vi "DP Waveform Averager PXI.vi"(0 "DataAcq":T3, 1 "DP Freqs":T2, 7 "iLevel":i32, 11 "error in":errorcluster, 12 "Abort":refnum<vi>, 13 "Reject Ref":T1) -> (4 "Error?":bool, 6 "Ave Wave":dbl[](graph), 8 "Averaged Spectrum (Vrms)":dbl[](array[numeric]), 10 "Phase spectrum":dbl[](array[numeric]), 14 "waveform cluster":cluster{i32, "dx":dbl, "Array":dbl[]}, 15 "error out":errorcluster)   [LabVIEW 2020]
uses:
  afcfbcde-8fef-4170-88b9-8379dbc42e1a.vi
  Typedefs/DP-Runtime State.ctl
  Typedefs/DP-Freqs.ctl
  Typedefs/DP-Rejection Settings.ctl
  Typedefs/DP-Rejection Settings Refnum.ctl
panel:
  out "# Spectra":i32
  out "# Waves":i32
  out "Spectrum":cluster{dbl, "dx":dbl, "Y":dbl[]}(graph)
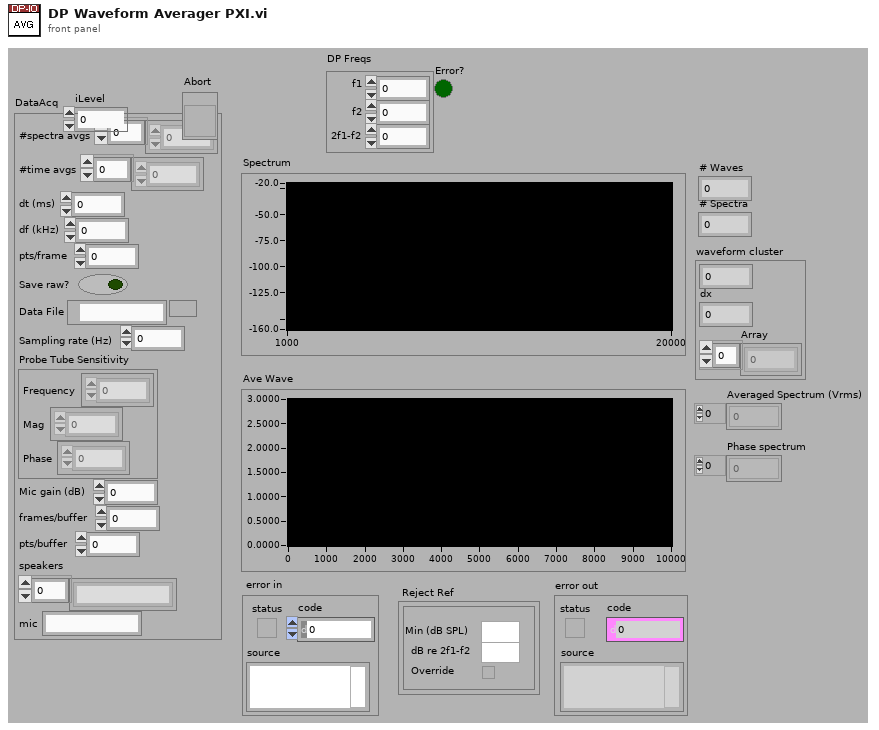
[diagram p1: front panel]
types:
  T1 = typedef "DP-Rejection Settings Refnum.ctl" = refnum<vi>
  T2 = typedef "DP-Freqs.ctl" = cluster{"f1":dbl, "f2":dbl, "2f1-f2":dbl}
  T3 = typedef "DP-Runtime State.ctl" = cluster{"#spectra avgs":i32[], "#time avgs":i32[], "dt (ms)":dbl, "df (kHz)":dbl, "pts/frame":i32, "Save raw?":bool, "Data File":path, "Sampling rate (Hz)":dbl, "Probe Tube Sensitivity":cluster{"Frequency":dbl[], "Mag":dbl[], "Phase":dbl[]}, "Mic gain (dB)":dbl, "frames/buffer":i32, "pts/buffer":i32, "speakers":string[], "mic":string}
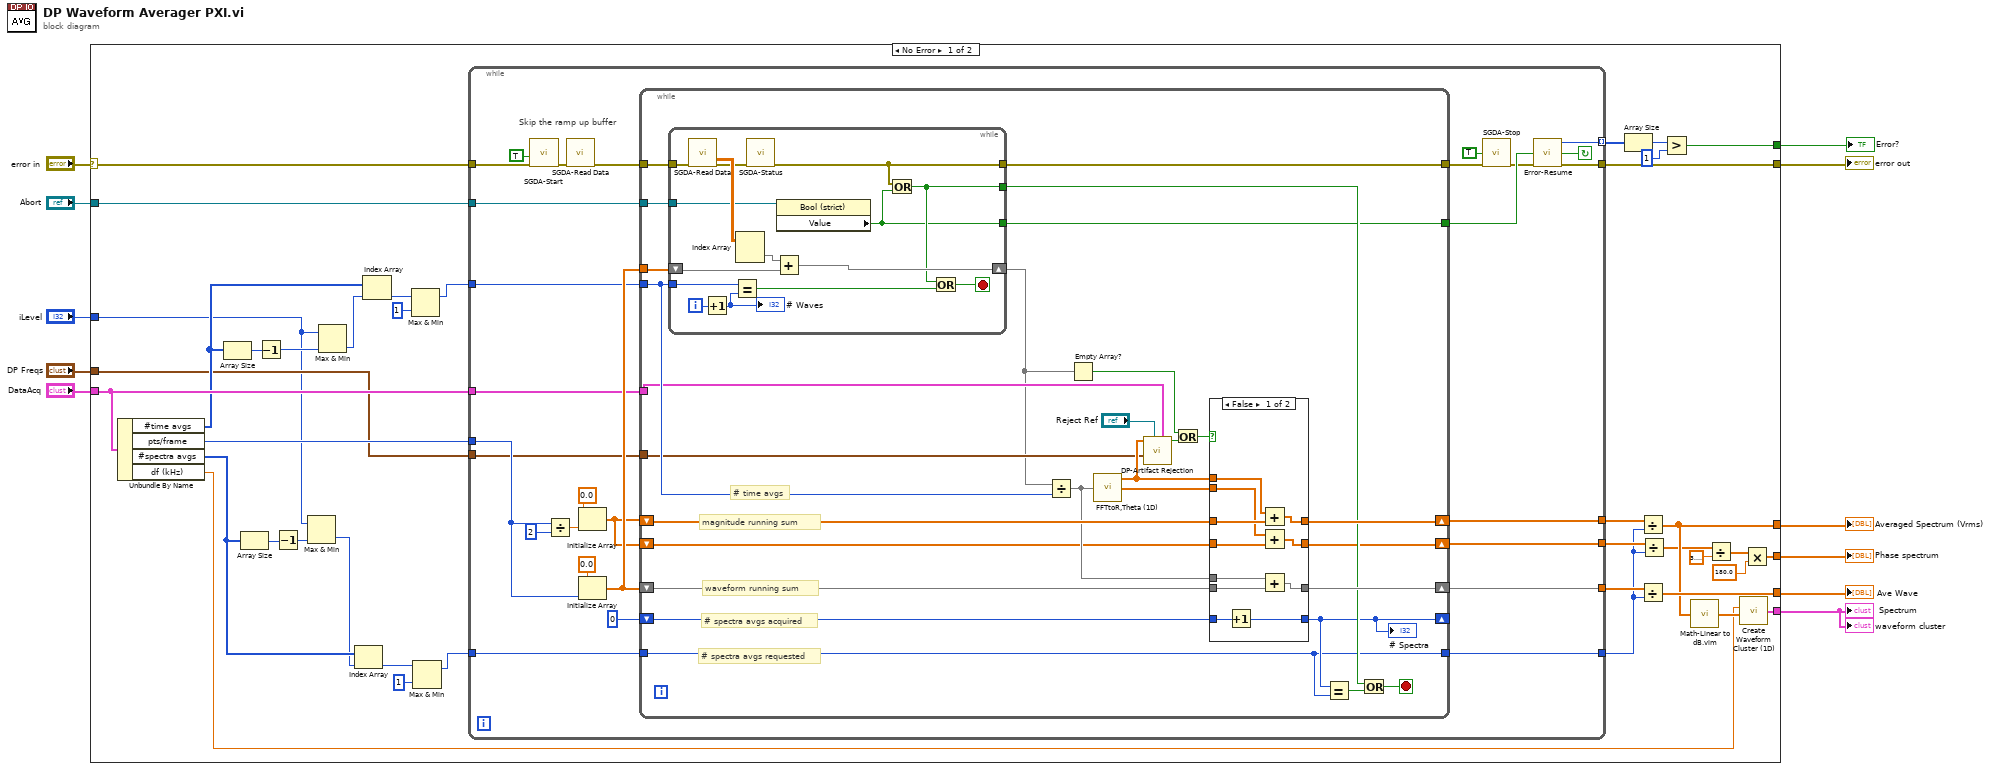
[diagram p0: block diagram]
diagram:
  n1 = case shown="No Error" "error in" {
    selector: "error in" -> [w28 w137]
    tunnel: [w48 _] -> w11
    tunnel: [w47 _] -> w10
    tunnel: [w43 _] -> w9
    tunnel: "Abort" -> [w42 _]
    tunnel: [w37 _] -> w7
    tunnel: "DataAcq" -> [w34 _]
    tunnel: [w33 w137] -> w5
    tunnel: [w29 _] -> w4
    tunnel: "iLevel" -> [w19 _]
    tunnel: "DP Freqs" -> [w21 _]
    frame No Error {
      n2 = Unbundle By Name(w34) -> ("#time avgs"=w27:i32[], "pts/frame"=w45:i32, "#spectra avgs"=w20:i32[], "df (kHz)"=w44:dbl)
      n3 = Array Size(array=w27) -> (size(s)=w26:i32)
      n4 = Array Size(array=w20) -> (size(s)=w23:i32)
      n5 = Decrement(x=w26) -> (x-1=w25:i32)
      n6 = Decrement(x=w23) -> (x-1=w22:i32)
      n7 = Max & Min(x=w19, y=w22) -> (min(x,y)=w18:i32)  [unwired: 1 out]
      n8 = Max & Min(x=w19, y=w25) -> (min(x,y)=w24:i32)  [unwired: 1 out]
      n9 = Index Array(array=w20, index=w18) -> (element=w13:i32)
      n10 = Index Array(array=w27, index=w24) -> (element=w17:i32)
      n11 = Max & Min(x=w17, y=1) -> (max(x,y)=w16:i32)  [unwired: 1 out]
      n12 = Max & Min(x=w13, y=1) -> (max(x,y)=w12:i32)  [unwired: 1 out]
      n13 = while {
        tunnel: [w78] -> w50
        tunnel: [w76] -> w49
        tunnel: [w56] -> w33
        tunnel: w16 -> [w70]
        tunnel: w45 -> [w69]
        tunnel: w42 -> [w68]
        tunnel: w28 -> [w67]
        tunnel: [w62] -> w41
        tunnel: w12 -> [w60]
        tunnel: [w59] -> w35
        tunnel: w21 -> [w58]
        tunnel: w34 -> [w57]
        tunnel: [w53] -> w32 mode=indexing
        stop <- w55 continue-if-true
        # "Skip the ramp up buffer"
        n14 = call "SGDA-Start.vi"("error in (no error)"=w67, "wait for DAQ? (F)"=TRUE) -> ("error out"=w65:errorcluster)  [unwired: 5 in]
        n15 = Divide(x=w69, y=2) -> (x/y=w71:dbl)
        n16 = call "SGDA-Read Data.vi"("error in (no error)"=w65) -> ("error out"=w66:errorcluster)  [unwired: 13 in, 1 out]
        n17 = Initialize Array(0.0, w71) -> (w63:dbl[])
        n18 = Initialize Array(0.0, w69) -> (w74:dbl[])
        n19 = while {
          tunnel: w70 -> [w100]
          shift-right: [w105] -> w78
          shift-left: w63 -> [w106]
          shift-right: [w103] -> w76
          shift-left: w74 -> [w104]
          tunnel: w74 -> [w101]
          tunnel: w66 -> [w102]
          tunnel: [w82] -> w75
          tunnel: w68 -> [w95]
          shift-right: [w94] -> w62
          shift-left: w63 -> [w92]
          shift-right: [w88] -> _
          shift-left: 0 -> [w89]
          tunnel: w60 -> [w87]
          tunnel: [w87] -> w59
          tunnel: w58 -> [w86]
          tunnel: w57 -> [w84]
          tunnel: [w83] -> w54
          stop <- w97 stop-if-true
          # "# spectra avgs acquired"
          # "# spectra avgs requested"
          # "# time avgs"
          # "waveform running sum"
          # "magnitude running sum"
          n20 = while {
            shift-right: [w133] -> w80
            shift-left: w101 -> [w134]
            tunnel: w100 -> [w132]
            tunnel: [w126] -> w98
            tunnel: w102 -> [w135]
            tunnel: [w122] -> w82
            tunnel: w95 -> [w125]
            tunnel: [w124] -> w83
            i -> [w131]
            stop <- w128 stop-if-true
            n21 = call "SGDA-Read Data.vi"("error in (no error)"=w135) -> ("AI Waveforms"=w136:dbl[][], "error out"=w123:errorcluster)  [unwired: 13 in]
            n22 = Increment(x=w131) -> (x+1=w130:i32)
            "# Waves" <- w130
            n23 = Equal?(x=w132, y=w130) -> (x = y?=w127:bool)
            n24 = Index Array(array=w136) -> (element=w129:dbl[])  [unwired: 2 in]
            n25 = call "SGDA-Status.vi"("error in (no error)"=w123) -> ("error out"=w122:errorcluster)  [unwired: 14 in]
            n26 = Add(x=w129, y=w134) -> (x+y=w133:dbl[])
            n27 = property class="Bool (strict)"(reference=w125) -> ("Value"=w124:bool)  [unwired: 1 in, 2 out]
            n28 = Or(x=w122, y=w124) -> (x .or. y?=w126:bool)
            n29 = Or(x=w126, y=w127) -> (x .or. y?=w128:bool)
          }
          n30 = Divide(x=w80, y=w100) -> (x/y=w99:dbl[])
          n31 = Empty Array?(array=w80) -> (empty?=w79:bool)
          n32 = call "FFTtoR,Theta (1D).VI"("X"=w99) -> ("+Freq. Mag of FFT"=w91:dbl[], "+Freq Theta of FFT"=w93:dbl[])  [unwired: 1 in]
          n33 = call "DP-Artifact Rejection.vi"("DataAcq"=w84, "Reject Ref"="Reject Ref", "DP Freqs"=w86, "Magnitude (Vrms)"=w91) -> ("Reject?"=w90:bool)  [unwired: 7 in]
          n34 = Or(x=w79, y=w90) -> (x .or. y?=w81:bool)
          n35 = case shown="False" w81 {
            tunnel: w106 -> [w117 w121]
            tunnel: [w116 w121] -> w105
            tunnel: w104 -> [w115 w119]
            tunnel: [w114 w119] -> w103
            tunnel: w99 -> [w113 _]
            tunnel: [w112 w120] -> w94
            tunnel: w93 -> [w111 _]
            tunnel: w92 -> [w110 w120]
            tunnel: w91 -> [w109 _]
            tunnel: w89 -> [w108 w118]
            tunnel: [w107 w118] -> w88
            frame False {
              n36 = Increment(x=w108) -> (x+1=w107:i32)
              n37 = Add(x=w109, y=w117) -> (x+y=w116:dbl[])
              n38 = Add(x=w111, y=w110) -> (x+y=w112:dbl[])
              n39 = Add(x=w113, y=w115) -> (x+y=w114:dbl[])
            }
            frame True {
            }
          }
          "# Spectra" <- w88
          n40 = Equal?(x=w88, y=w87) -> (x = y?=w96:bool)
          n41 = Or(x=w98, y=w96) -> (x .or. y?=w97:bool)
        }
        n42 = call "SGDA-Stop.vi"("Clear ActiveX (F)"=TRUE, "error in (no error)"=w75) -> ("error out"=w52:errorcluster)  [unwired: 13 in]
        n43 = call "Error-Resume.vi"("Abort"=w54, "error in (no error)"=w52) -> ("code"=w53:i32, "Resume?"=w55:bool, "error out"=w56:errorcluster)  [unwired: 11 in]
      }
      n44 = Array Size(array=w32) -> (size(s)=w31:i32)
      n45 = Divide(x=w50, y=w35) -> (x/y=w47:dbl[])
      n46 = Divide(x=w49, y=w35) -> (x/y=w48:dbl[])
      n47 = Divide(x=w41, y=w35) -> (x/y=w40:dbl[])
      n48 = Greater?(x=w31, y=1) -> (0:w29:bool)
      n49 = call "Math-Linear to dB.vim"("linear"=w47) -> ("dB"=w46:dbl[])
      n50 = Divide(x=w40, y=3.141592653589793) -> (x/y=w39:dbl[])
      n51 = call "Create Waveform Cluster (1D).vi"("dx"=w44, "Y"=w46) -> ("waveform cluster"=w43:cluster{dbl, "dx":dbl, "Y":dbl[]})  [unwired: 3 in]
      n52 = Multiply(x=w39, y=180.0) -> (x*y=w37:dbl[])
    }
    frame Error {
    }
  }
  "Spectrum" <- w9
  "Ave Wave" <- w11
  "error out" <- w5
  "waveform cluster" <- w9
  "Averaged Spectrum (Vrms)" <- w10
  "Phase spectrum" <- w7
  "Error?" <- w4
